vi "String.Split String to 1D Array.vi"(7 "Remove Empty Strings":bool, 10 "Delimiter":string=",", 11 "String":string) -> (3 "Items":string[](array[string]))   [LabVIEW 2019]
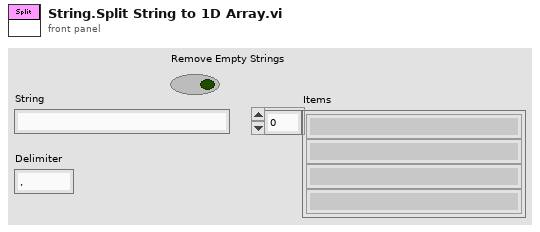
[diagram p1: front panel]
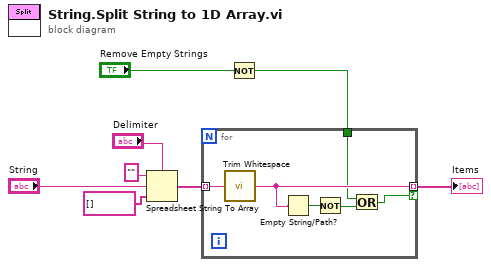
[diagram p0: block diagram]
diagram:
  n1 = Spreadsheet String To Array(delimiter (Tab)="Delimiter", format string="", spreadsheet string="String", array type (2D Dbl)=string[] [] ("format string")) -> (array=w4:string[])
  n2 = Not(x="Remove Empty Strings") -> (.not. x?=w1:bool)
  n3 = for {
    tunnel: w4 -> [w14] mode=indexing
    tunnel: [w13] -> w3 mode=indexing if=w10
    tunnel: w1 -> [w9]
    n4 = call <vilib>:"Trim Whitespace.vi"("string"=w14) -> ("trimmed string"=w13:string)  [unwired: 1 in]
    n5 = Empty String/Path?(string/path=w13) -> (empty?=w12:bool)
    n6 = Not(x=w12) -> (.not. x?=w11:bool)
    n7 = Or(x=w9, y=w11) -> (x .or. y?=w10:bool)
  }
  "Items" <- w3
